vi "XML Write.vi"(7 "XML File Path Write":path=path "c:/config.xml", 8 "Error In":errorcluster, 11 "FOFB Parameters":T1) -> (0 "Error Out":errorcluster, 3 "XML File Path Out":path)   [LabVIEW 2011, in "XML VIs.lvlib"]
uses:
  XML VIs.lvlib
  Types Definitions/Type FOFB Parameters.ctl
  Types Definitions/Type Network Configuration.ctl
  Types Definitions/Type FA Configuration.ctl
  Types Definitions/Type Response Matrix Measurement Configuration.ctl
  Types Definitions/Type Correction Algorithm Configuration.ctl
  Types Definitions/Type Acquisition Network Configuration.ctl
  Types Definitions/Type Actuation Network Configuration.ctl
  Third Party/GXML/GXML.lvlib
  Type Definitions.lvlib
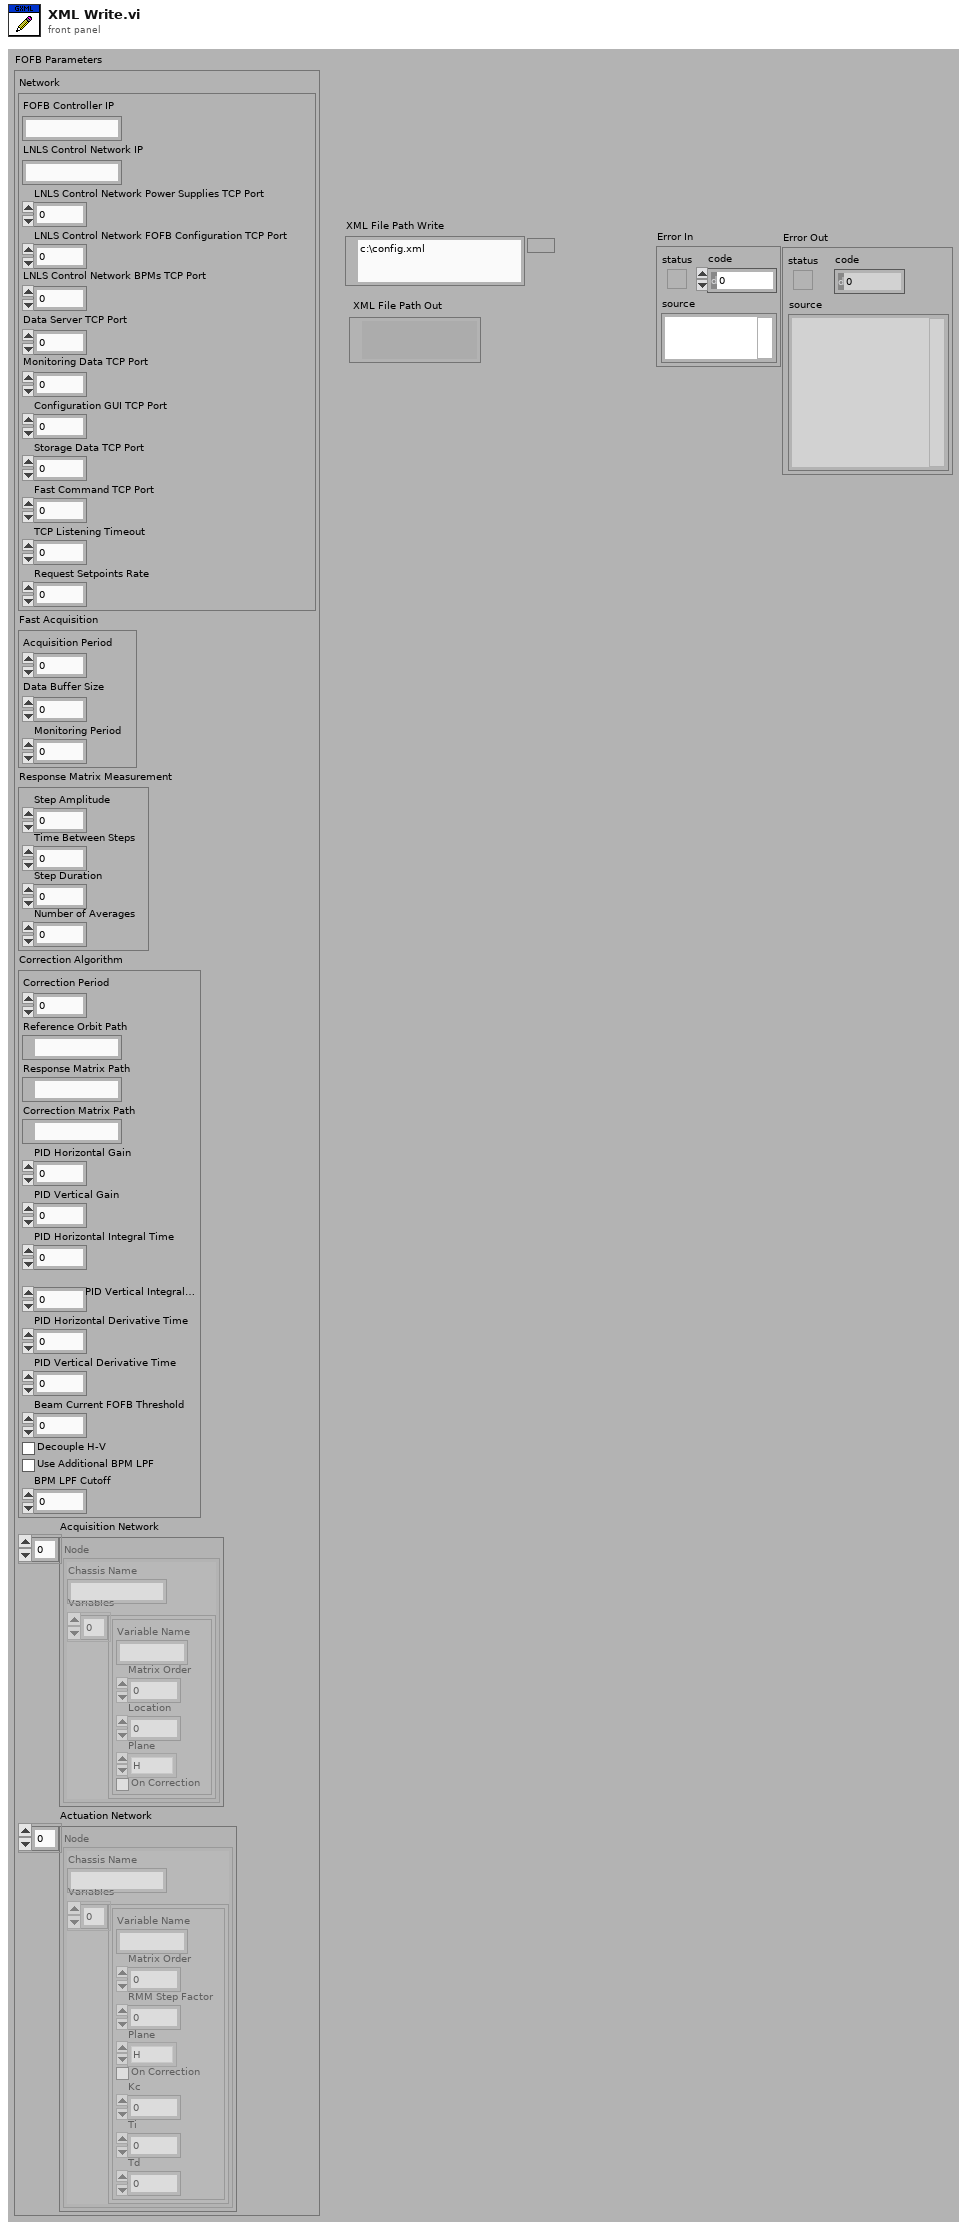
[diagram p1: front panel]
types:
  T1 = typedef "Type Definitions.lvlib/Type FOFB Parameters.ctl" = cluster{"Network":T2, "Fast Acquisition":T3, "Response Matrix Measurement":T4, "Correction Algorithm":T5, "Acquisition Network":T6, "Actuation Network":T7}
  T2 = typedef "Type Definitions.lvlib/Type Network Configuration.ctl" = cluster{"FOFB Controller IP":string, "LNLS Control Network IP":string, "LNLS Control Network Power Supplies TCP Port":u16, "LNLS Control Network FOFB Configuration TCP Port":u16, "LNLS Control Network BPMs TCP Port":u16, "Data Server TCP Port":u16, "Monitoring Data TCP Port":u16, "Configuration GUI TCP Port":u16, "Storage Data TCP Port":u16, "Fast Command TCP Port":u16, "TCP Listening Timeout":i32, "Request Setpoints Rate":u16}
  T3 = typedef "Type Definitions.lvlib/Type FA Configuration.ctl" = cluster{"Acquisition Period":u32, "Data Buffer Size":u32, "Monitoring Period":u32}
  T4 = typedef "Type Definitions.lvlib/Type Response Matrix Measurement Configuration.ctl" = cluster{"Step Amplitude":dbl, "Time Between Steps":u32, "Step Duration":u32, "Number of Averages":u32}
  T5 = typedef "Type Definitions.lvlib/Type Correction Algorithm Configuration.ctl" = cluster{"Correction Period":u32, "Reference Orbit Path":path, "Response Matrix Path":path, "Correction Matrix Path":path, "PID Horizontal Gain":dbl, "PID Vertical Gain":dbl, "PID Horizontal Integral Time":dbl, "PID Vertical Integral Time":dbl, "PID Horizontal Derivative Time":dbl, "PID Vertical Derivative Time":dbl, "Beam Current FOFB Threshold":dbl, "Decouple H-V":bool, "Use Additional BPM LPF":bool, "BPM LPF Cutoff":dbl}
  T6 = typedef "Type Definitions.lvlib/Type Acquisition Network Configuration.ctl" = cluster{"Chassis Name":string, "Variables":cluster{"Variable Name":string, "Matrix Order":u32, "Location":dbl, "Plane":enum8{"H", "V"}, "On Correction":bool}[]}[]
  T7 = typedef "Type Definitions.lvlib/Type Actuation Network Configuration.ctl" = cluster{"Chassis Name":string, "Variables":cluster{"Variable Name":string, "Matrix Order":u32, "RMM Step Factor":dbl, "Plane":enum8{"H", "V"}, "On Correction":bool, "Kc":dbl, "Ti":dbl, "Td":dbl}[]}[]
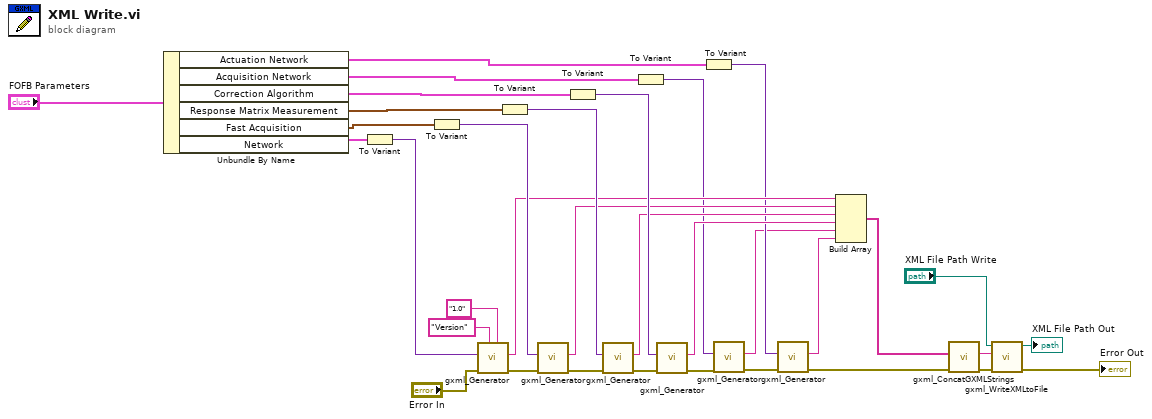
[diagram p0: block diagram]
diagram:
  n1 = Unbundle By Name("FOFB Parameters") -> ("Actuation Network"=w1:T7, "Acquisition Network"=w2:T6, "Correction Algorithm"=w3:T5, "Response Matrix Measurement"=w4:T4, "Fast Acquisition"=w5:T3, "Network"=w6:T2)
  n2 = To Variant(anything=w6) -> (Variant=w18:variant)
  n3 = To Variant(anything=w5) -> (Variant=w17:variant)
  n4 = call "gxml_Generator.vi"("Version String"="1.0", "Version Tag Name"="Version", "error in"="Error In", "Variant"=w18) -> ("error out"=w19:errorcluster, "XML String Out"=w15:string)  [unwired: 6 in]
  n5 = To Variant(anything=w4) -> (Variant=w21:variant)
  n6 = call "gxml_Generator.vi"("error in"=w19, "Variant"=w17) -> ("error out"=w22:errorcluster, "XML String Out"=w16:string)  [unwired: 8 in]
  n7 = To Variant(anything=w3) -> (Variant=w27:variant)
  n8 = call "gxml_Generator.vi"("error in"=w22, "Variant"=w21) -> ("error out"=w20:errorcluster, "XML String Out"=w23:string)  [unwired: 8 in]
  n9 = To Variant(anything=w2) -> (Variant=w12:variant)
  n10 = call "gxml_Generator.vi"("error in"=w20, "Variant"=w27) -> ("error out"=w10:errorcluster, "XML String Out"=w26:string)  [unwired: 8 in]
  n11 = To Variant(anything=w1) -> (Variant=w11:variant)
  n12 = call "gxml_Generator.vi"("error in"=w10, "Variant"=w12) -> ("error out"=w14:errorcluster, "XML String Out"=w9:string)  [unwired: 8 in]
  n13 = call "gxml_Generator.vi"("error in"=w14, "Variant"=w11) -> ("error out"=w13:errorcluster, "XML String Out"=w8:string)  [unwired: 8 in]
  n14 = Build Array(w15, w16, w23, w26, w9, w8) -> (w32:string[])
  n15 = call "gxml_ConcatGXMLStrings.vi"("error in"=w13, "GXML Strings"=w32) -> ("error out"=w33:errorcluster, "Concatenated GXML String"=w34:string)  [unwired: 8 in]
  n16 = call "gxml_WriteXMLtoFile.vi"("error in"=w33, "XML Input"=w34, "XML File Path"="XML File Path Write") -> ("error out"=→"Error Out":errorcluster, "XML File Path Out"=→"XML File Path Out":path)  [unwired: 7 in]
